vi "HandleObservationSync_003.vi"(8 "error in (no error)":errorcluster, 11 "S4GUI in":refnum<class "S4GUI.lvclass">) -> (0 "error out":errorcluster, 3 "S4GUI out":refnum<class "S4GUI.lvclass">)   [LabVIEW 2018, in "S4GUI.lvclass"] (continued)
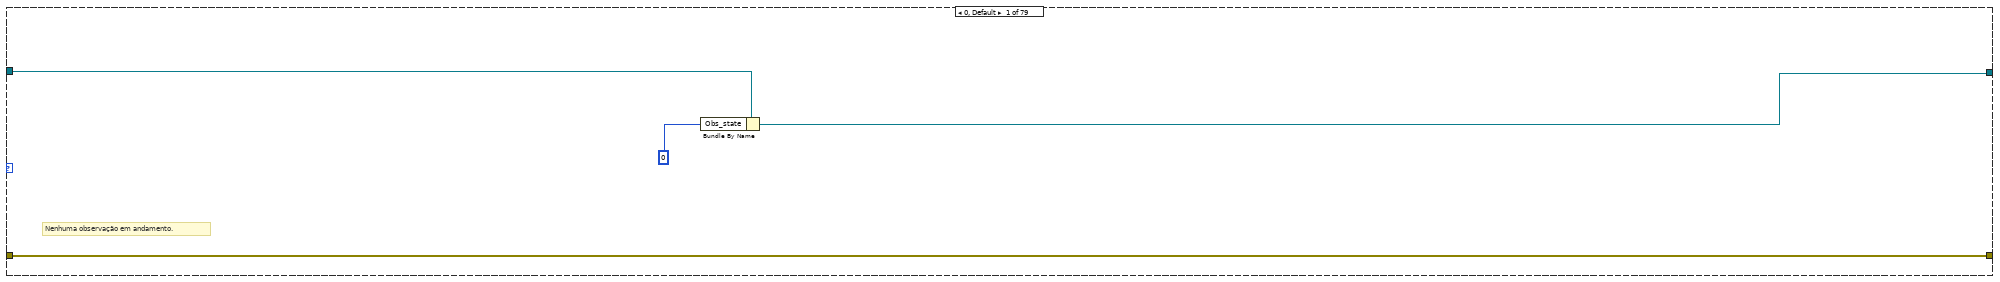
[diagram p2: hidden frame]
          n1819 = Increment(x=w5017) -> (x+1=w5016:u32)
          n1820 = Bundle By Name(cluster=w4999, "Obs_state"=w5016) -> (w5015:refnum<class "S4GUI.lvclass">)
        }
        frame 363 {
          # "T: mode EXPOSE\nF: mode FIRE\nNa seq de foco, só \ndeve usar mode EXPOSE."
          # "Espera todos os canais chegarem ao estado de repouso.\n(estado 0  de Channel:Run.vi)."
          n1821 = call-dynamic "Read AcquisitionA.vi"("error in (no error)"=w5143, "S4ACS_GUI in"=w5144) -> ("error out"=w5122:errorcluster, "Acquisition.lvclass"=w5123:refnum<class "Acquisition.lvclass">, "S4ACS_GUI out"=w5146:refnum<class "S4GUI.lvclass">)  [unwired: 7 in]
          n1822 = call-dynamic "Read enabled.vi"("error in (no error)"=w5122, "Server in"=w5123) -> ("error out"=w5124:errorcluster, "enabled"=w5126:bool, "Server out"=w5125:refnum<class "Acquisition.lvclass">)  [unwired: 7 in]
          n1823 = case shown="True" w5126 {
            tunnel: [w5220 w5238] -> w5147
            tunnel: [w5219 w5237] -> w5145
            tunnel: w5125 -> [w5220 w5230]
            tunnel: w5124 -> [w5219 w5229]
            tunnel: [TRUE w5222] -> w5103
            tunnel: [FALSE w5223] -> w5099
            frame False {
            }
            frame True {
              n1824 = call-dynamic "Read Channel.vi"("error in (no error)"=w5229, "Acquisition in"=w5230) -> ("error out"=w5226:errorcluster, "Channel.lvclass"=w5227:refnum<class "Channel.lvclass">, "Acquisition out"=w5239:refnum<class "Acquisition.lvclass">)  [unwired: 7 in]
              n1825 = call-dynamic "Read wait_expose.vi"("error in (no error)"=w5226, "Channel in"=w5227) -> ("error out"=w5224:errorcluster, "wait_expose"=w5223:bool, "Channel out"=w5225:refnum<class "Channel.lvclass">)  [unwired: 7 in]
              n1826 = call-dynamic "Read State Machine.vi"("error in (no error)"=w5224, "Device in"=w5225) -> ("error out"=w5231:errorcluster, "State Machine.lvclass"=w5233:refnum<class "State Machine.lvclass">, "Device out"=w5235:refnum<class "Channel.lvclass">)  [unwired: 7 in]
              n1827 = call-dynamic "Read State.vi"("error in (no error)"=w5231, "State Machine in"=w5233) -> ("error out"=w5228:errorcluster, "State"=w5221:i32, "State Machine out"=w5232:refnum<class "State Machine.lvclass">)  [unwired: 7 in]
              n1828 = Equal To 0?(x=w5221) -> (x = 0?=w5222:bool)
              n1829 = call-dynamic "Write State Machine.vi"("error in (no error)"=w5228, "State Machine.lvclass"=w5232, "Device in"=w5235) -> ("error out"=w5234:errorcluster, "Device out"=w5236:refnum<class "Channel.lvclass">)  [unwired: 7 in]
              n1830 = call-dynamic "Write Channel.vi"("error in (no error)"=w5234, "Channel.lvclass"=w5236, "Acquisition in"=w5239) -> ("error out"=w5237:errorcluster, "Acquisition out"=w5238:refnum<class "Acquisition.lvclass">)  [unwired: 7 in]
            }
          }
          n1831 = call-dynamic "Write AcquisitionA.vi"("error in (no error)"=w5145, "Acquisition.lvclass"=w5147, "S4ACS_GUI in"=w5146) -> ("error out"=w5139:errorcluster, "S4ACS_GUI out"=w5140:refnum<class "S4GUI.lvclass">)  [unwired: 7 in]
          n1832 = call "Read AcquisitionB.vi"("error in (no error)"=w5139, "S4ACS_GUI in"=w5140) -> ("error out"=w5119:errorcluster, "Acquisition.lvclass"=w5121:refnum<class "Acquisition.lvclass">, "S4ACS_GUI out"=w5137:refnum<class "S4GUI.lvclass">)  [unwired: 7 in]
          n1833 = call-dynamic "Read enabled.vi"("error in (no error)"=w5119, "Server in"=w5121) -> ("error out"=w5118:errorcluster, "enabled"=w5117:bool, "Server out"=w5120:refnum<class "Acquisition.lvclass">)  [unwired: 7 in]
          n1834 = case shown="True" w5117 {
            tunnel: w5120 -> [w5197 w5216]
            tunnel: w5118 -> [w5196 w5215]
            tunnel: [w5197 w5213] -> w5138
            tunnel: [w5196 w5212] -> w5136
            tunnel: [TRUE w5204] -> w5102
            tunnel: [FALSE ("expose") w5198] -> w5098
            frame False {
            }
            frame True {
              n1835 = call-dynamic "Read Channel.vi"("error in (no error)"=w5215, "Acquisition in"=w5216) -> ("error out"=w5200:errorcluster, "Channel.lvclass"=w5202:refnum<class "Channel.lvclass">, "Acquisition out"=w5214:refnum<class "Acquisition.lvclass">)  [unwired: 7 in]
              n1836 = call-dynamic "Read wait_expose.vi"("error in (no error)"=w5200, "Channel in"=w5202) -> ("error out"=w5199:errorcluster, "wait_expose"=w5198:bool, "Channel out"=w5201:refnum<class "Channel.lvclass">)  [unwired: 7 in]
              n1837 = call-dynamic "Read State Machine.vi"("error in (no error)"=w5199, "Device in"=w5201) -> ("error out"=w5206:errorcluster, "State Machine.lvclass"=w5208:refnum<class "State Machine.lvclass">, "Device out"=w5210:refnum<class "Channel.lvclass">)  [unwired: 7 in]
              n1838 = call-dynamic "Read State.vi"("error in (no error)"=w5206, "State Machine in"=w5208) -> ("error out"=w5205:errorcluster, "State"=w5203:i32, "State Machine out"=w5207:refnum<class "State Machine.lvclass">)  [unwired: 7 in]
              n1839 = Equal To 0?(x=w5203) -> (x = 0?=w5204:bool)
              n1840 = call-dynamic "Write State Machine.vi"("error in (no error)"=w5205, "State Machine.lvclass"=w5207, "Device in"=w5210) -> ("error out"=w5209:errorcluster, "Device out"=w5211:refnum<class "Channel.lvclass">)  [unwired: 7 in]
              n1841 = call-dynamic "Write Channel.vi"("error in (no error)"=w5209, "Channel.lvclass"=w5211, "Acquisition in"=w5214) -> ("error out"=w5212:errorcluster, "Acquisition out"=w5213:refnum<class "Acquisition.lvclass">)  [unwired: 7 in]
            }
          }
          n1842 = call "Write AcquisitionB.vi"("error in (no error)"=w5136, "Acquisition.lvclass"=w5138, "S4ACS_GUI in"=w5137) -> ("error out"=w5132:errorcluster, "S4ACS_GUI out"=w5131:refnum<class "S4GUI.lvclass">)  [unwired: 7 in]
          n1843 = call-dynamic "Read AcquisitionC.vi"("error in (no error)"=w5132, "S4ACS_GUI in"=w5131) -> ("error out"=w5114:errorcluster, "Acquisition.lvclass"=w5116:refnum<class "Acquisition.lvclass">, "S4ACS_GUI out"=w5134:refnum<class "S4GUI.lvclass">)  [unwired: 7 in]
          n1844 = call-dynamic "Read enabled.vi"("error in (no error)"=w5114, "Server in"=w5116) -> ("error out"=w5113:errorcluster, "enabled"=w5112:bool, "Server out"=w5115:refnum<class "Acquisition.lvclass">)  [unwired: 7 in]
          n1845 = case shown="True" w5112 {
            tunnel: [w5173 w5188] -> w5135
            tunnel: [w5174 w5187] -> w5133
            tunnel: w5115 -> [w5174 w5183]
            tunnel: w5113 -> [w5173 w5182]
            tunnel: [TRUE w5180] -> w5101
            tunnel: [FALSE ("expose") w5175] -> w5097
            frame False {
            }
            frame True {
              n1846 = call-dynamic "Read Channel.vi"("error in (no error)"=w5182, "Acquisition in"=w5183) -> ("error out"=w5177:errorcluster, "Channel.lvclass"=w5179:refnum<class "Channel.lvclass">, "Acquisition out"=w5186:refnum<class "Acquisition.lvclass">)  [unwired: 7 in]
              n1847 = call-dynamic "Read wait_expose.vi"("error in (no error)"=w5177, "Channel in"=w5179) -> ("error out"=w5176:errorcluster, "wait_expose"=w5175:bool, "Channel out"=w5178:refnum<class "Channel.lvclass">)  [unwired: 7 in]
              n1848 = call-dynamic "Read State Machine.vi"("error in (no error)"=w5176, "Device in"=w5178) -> ("error out"=w5184:errorcluster, "State Machine.lvclass"=w5192:refnum<class "State Machine.lvclass">, "Device out"=w5190:refnum<class "Channel.lvclass">)  [unwired: 7 in]
              n1849 = call-dynamic "Read State.vi"("error in (no error)"=w5184, "State Machine in"=w5192) -> ("error out"=w5185:errorcluster, "State"=w5181:i32, "State Machine out"=w5193:refnum<class "State Machine.lvclass">)  [unwired: 7 in]
              n1850 = Equal To 0?(x=w5181) -> (x = 0?=w5180:bool)
              n1851 = call-dynamic "Write State Machine.vi"("error in (no error)"=w5185, "State Machine.lvclass"=w5193, "Device in"=w5190) -> ("error out"=w5191:errorcluster, "Device out"=w5189:refnum<class "Channel.lvclass">)  [unwired: 7 in]
              n1852 = call-dynamic "Write Channel.vi"("error in (no error)"=w5191, "Channel.lvclass"=w5189, "Acquisition in"=w5186) -> ("error out"=w5188:errorcluster, "Acquisition out"=w5187:refnum<class "Acquisition.lvclass">)  [unwired: 7 in]
            }
          }
          n1853 = call-dynamic "Write AcquisitionC.vi"("error in (no error)"=w5135, "Acquisition.lvclass"=w5133, "S4ACS_GUI in"=w5134) -> ("error out"=w5111:errorcluster, "S4ACS_GUI out"=w5127:refnum<class "S4GUI.lvclass">)  [unwired: 7 in]
          n1854 = call-dynamic "Read AcquisitionD.vi"("error in (no error)"=w5111, "S4ACS_GUI in"=w5127) -> ("error out"=w5107:errorcluster, "Acquisition.lvclass"=w5110:refnum<class "Acquisition.lvclass">, "S4ACS_GUI out"=w5129:refnum<class "S4GUI.lvclass">)  [unwired: 7 in]
          n1855 = call-dynamic "Read enabled.vi"("error in (no error)"=w5107, "Server in"=w5110) -> ("error out"=w5108:errorcluster, "enabled"=w5106:bool, "Server out"=w5109:refnum<class "Acquisition.lvclass">)  [unwired: 7 in]
          n1856 = case shown="True" w5106 {
            tunnel: [w5151 w5169] -> w5130
            tunnel: [w5150 w5168] -> w5128
            tunnel: [TRUE w5158] -> w5100
            tunnel: w5109 -> [w5151 w5160]
            tunnel: w5108 -> [w5150 w5159]
            tunnel: [FALSE ("expose") w5152] -> w5096
            frame False {
            }
            frame True {
              n1857 = call-dynamic "Read Channel.vi"("error in (no error)"=w5159, "Acquisition in"=w5160) -> ("error out"=w5154:errorcluster, "Channel.lvclass"=w5156:refnum<class "Channel.lvclass">, "Acquisition out"=w5170:refnum<class "Acquisition.lvclass">)  [unwired: 7 in]
              n1858 = call-dynamic "Read wait_expose.vi"("error in (no error)"=w5154, "Channel in"=w5156) -> ("error out"=w5153:errorcluster, "wait_expose"=w5152:bool, "Channel out"=w5155:refnum<class "Channel.lvclass">)  [unwired: 7 in]
              n1859 = call-dynamic "Read State Machine.vi"("error in (no error)"=w5153, "Device in"=w5155) -> ("error out"=w5162:errorcluster, "State Machine.lvclass"=w5164:refnum<class "State Machine.lvclass">, "Device out"=w5166:refnum<class "Channel.lvclass">)  [unwired: 7 in]
              n1860 = call-dynamic "Read State.vi"("error in (no error)"=w5162, "State Machine in"=w5164) -> ("error out"=w5161:errorcluster, "State"=w5157:i32, "State Machine out"=w5163:refnum<class "State Machine.lvclass">)  [unwired: 7 in]
              n1861 = Equal To 0?(x=w5157) -> (x = 0?=w5158:bool)
              n1862 = call-dynamic "Write State Machine.vi"("error in (no error)"=w5161, "State Machine.lvclass"=w5163, "Device in"=w5166) -> ("error out"=w5165:errorcluster, "Device out"=w5167:refnum<class "Channel.lvclass">)  [unwired: 7 in]
              n1863 = call-dynamic "Write Channel.vi"("error in (no error)"=w5165, "Channel.lvclass"=w5167, "Acquisition in"=w5170) -> ("error out"=w5168:errorcluster, "Acquisition out"=w5169:refnum<class "Acquisition.lvclass">)  [unwired: 7 in]
            }
          }
          n1864 = call-dynamic "Write AcquisitionD.vi"("error in (no error)"=w5128, "Acquisition.lvclass"=w5130, "S4ACS_GUI in"=w5129) -> ("error out"=w5094:errorcluster, "S4ACS_GUI out"=w5095:refnum<class "S4GUI.lvclass">)  [unwired: 7 in]
          n1865 = Compound Arithmetic op=OR(w5099, w5098, w5097, w5096) -> ()  [unwired: 1 out]
          n1866 = Compound Arithmetic op=AND(w5103, w5102, w5101, w5100) -> (w5104:bool)
          n1867 = Increment(x=w5105) -> (x+1=w5093:u32)
          n1868 = Select(t=w5093, s=w5104, f=w5105) -> (s? t:f=w5141:u32)
          n1869 = Bundle By Name(cluster=w5095, "Obs_state"=w5141) -> (w5142:refnum<class "S4GUI.lvclass">)
        }
        frame 364 {
          n1870 = flat-sequence {
            tunnel: [w5253] -> w5241
            tunnel: w5242 -> [w5253]
            tunnel: [w5249] -> w5240
            frame #0 {
              # "Espera 2s desde que enviou o comando\nWRITE_HEADER_DATA para os ACS"
              n1871 = local read "time9"() -> (w5248:u32)
              n1872 = Tick Count (ms)() -> (millisecond timer value=w5252:u32)
              "time 10" <- w5252
              n1873 = Subtract(x=w5252, y=w5248) -> (x-y=w5251:u32)
              "delay 89" <- w5251
              n1874 = Greater?(x=w5251, y=u32 2000) -> (0:w5249:bool)
            }
          }
          n1875 = Increment(x=w5245) -> (x+1=w5244:u32)
          n1876 = Select(t=w5244, s=w5240, f=w5245) -> (s? t:f=w5246:u32)
          n1877 = Bundle By Name(cluster=w5243, "Obs_state"=w5246) -> (w5247:refnum<class "S4GUI.lvclass">)
        }
        frame 365 {
          n1878 = call-dynamic "Read AcquisitionA.vi"("error in (no error)"=w5294, "S4ACS_GUI in"=w5295) -> ("error out"=w5270:errorcluster, "Acquisition.lvclass"=w5273:refnum<class "Acquisition.lvclass">, "S4ACS_GUI out"=w5297:refnum<class "S4GUI.lvclass">)  [unwired: 7 in]
          n1879 = call-dynamic "Read enabled.vi"("error in (no error)"=w5270, "Server in"=w5273) -> ("error out"=w5269:errorcluster, "enabled"=w5271:bool, "Server out"=w5272:refnum<class "Acquisition.lvclass">)  [unwired: 7 in]
          n1880 = case shown="True" w5271 {
            tunnel: w5272 -> [w5351 w5366]
            tunnel: w5269 -> [w5350 w5365]
            tunnel: [w5351 w5363] -> w5298
            tunnel: [w5350 w5362] -> w5296
            frame False {
            }
            frame True {
              n1881 = call-dynamic "Read Channel.vi"("error in (no error)"=w5365, "Acquisition in"=w5366) -> ("error out"=w5358:errorcluster, "Channel.lvclass"=w5357:refnum<class "Channel.lvclass">, "Acquisition out"=w5364:refnum<class "Acquisition.lvclass">)  [unwired: 7 in]
              n1882 = call-dynamic "Read State Machine.vi"("error in (no error)"=w5358, "Device in"=w5357) -> ("error out"=w5359:errorcluster, "State Machine.lvclass"=w5361:refnum<class "State Machine.lvclass">, "Device out"=w5355:refnum<class "Channel.lvclass">)  [unwired: 7 in]
              n1883 = call "Next State.vi"("error in (no error)"=w5359, "New_State"=50, "State Machine in"=w5361) -> ("error out"=w5352:errorcluster, "State Machine out"=w5353:refnum<class "State Machine.lvclass">)  [unwired: 7 in]
              n1884 = call-dynamic "Write State Machine.vi"("error in (no error)"=w5352, "State Machine.lvclass"=w5353, "Device in"=w5355) -> ("error out"=w5354:errorcluster, "Device out"=w5356:refnum<class "Channel.lvclass">)  [unwired: 7 in]
              n1885 = call-dynamic "Write Channel.vi"("error in (no error)"=w5354, "Channel.lvclass"=w5356, "Acquisition in"=w5364) -> ("error out"=w5362:errorcluster, "Acquisition out"=w5363:refnum<class "Acquisition.lvclass">)  [unwired: 7 in]
            }
          }
          n1886 = call-dynamic "Write AcquisitionA.vi"("error in (no error)"=w5296, "Acquisition.lvclass"=w5298, "S4ACS_GUI in"=w5297) -> ("error out"=w5289:errorcluster, "S4ACS_GUI out"=w5290:refnum<class "S4GUI.lvclass">)  [unwired: 7 in]
          n1887 = call "Read AcquisitionB.vi"("error in (no error)"=w5289, "S4ACS_GUI in"=w5290) -> ("error out"=w5266:errorcluster, "Acquisition.lvclass"=w5268:refnum<class "Acquisition.lvclass">, "S4ACS_GUI out"=w5287:refnum<class "S4GUI.lvclass">)  [unwired: 7 in]
          n1888 = call-dynamic "Read enabled.vi"("error in (no error)"=w5266, "Server in"=w5268) -> ("error out"=w5265:errorcluster, "enabled"=w5264:bool, "Server out"=w5267:refnum<class "Acquisition.lvclass">)  [unwired: 7 in]
          n1889 = case shown="True" w5264 {
            tunnel: w5267 -> [w5334 w5349]
            tunnel: w5265 -> [w5333 w5348]
            tunnel: [w5334 w5346] -> w5288
            tunnel: [w5333 w5345] -> w5286
            frame False {
            }
            frame True {
              n1890 = call-dynamic "Read Channel.vi"("error in (no error)"=w5348, "Acquisition in"=w5349) -> ("error out"=w5341:errorcluster, "Channel.lvclass"=w5340:refnum<class "Channel.lvclass">, "Acquisition out"=w5347:refnum<class "Acquisition.lvclass">)  [unwired: 7 in]
              n1891 = call-dynamic "Read State Machine.vi"("error in (no error)"=w5341, "Device in"=w5340) -> ("error out"=w5342:errorcluster, "State Machine.lvclass"=w5344:refnum<class "State Machine.lvclass">, "Device out"=w5338:refnum<class "Channel.lvclass">)  [unwired: 7 in]
              n1892 = call "Next State.vi"("error in (no error)"=w5342, "New_State"=50, "State Machine in"=w5344) -> ("error out"=w5335:errorcluster, "State Machine out"=w5336:refnum<class "State Machine.lvclass">)  [unwired: 7 in]
              n1893 = call-dynamic "Write State Machine.vi"("error in (no error)"=w5335, "State Machine.lvclass"=w5336, "Device in"=w5338) -> ("error out"=w5337:errorcluster, "Device out"=w5339:refnum<class "Channel.lvclass">)  [unwired: 7 in]
              n1894 = call-dynamic "Write Channel.vi"("error in (no error)"=w5337, "Channel.lvclass"=w5339, "Acquisition in"=w5347) -> ("error out"=w5345:errorcluster, "Acquisition out"=w5346:refnum<class "Acquisition.lvclass">)  [unwired: 7 in]
            }
          }
          n1895 = call "Write AcquisitionB.vi"("error in (no error)"=w5286, "Acquisition.lvclass"=w5288, "S4ACS_GUI in"=w5287) -> ("error out"=w5282:errorcluster, "S4ACS_GUI out"=w5281:refnum<class "S4GUI.lvclass">)  [unwired: 7 in]
          n1896 = call-dynamic "Read AcquisitionC.vi"("error in (no error)"=w5282, "S4ACS_GUI in"=w5281) -> ("error out"=w5261:errorcluster, "Acquisition.lvclass"=w5263:refnum<class "Acquisition.lvclass">, "S4ACS_GUI out"=w5284:refnum<class "S4GUI.lvclass">)  [unwired: 7 in]
          n1897 = call-dynamic "Read enabled.vi"("error in (no error)"=w5261, "Server in"=w5263) -> ("error out"=w5260:errorcluster, "enabled"=w5259:bool, "Server out"=w5262:refnum<class "Acquisition.lvclass">)  [unwired: 7 in]
          n1898 = case shown="True" w5259 {
            tunnel: [w5316 w5324] -> w5285
            tunnel: [w5317 w5323] -> w5283
            tunnel: w5262 -> [w5317 w5321]
            tunnel: w5260 -> [w5316 w5320]
            frame False {
            }
            frame True {
              n1899 = call-dynamic "Read Channel.vi"("error in (no error)"=w5320, "Acquisition in"=w5321) -> ("error out"=w5328:errorcluster, "Channel.lvclass"=w5329:refnum<class "Channel.lvclass">, "Acquisition out"=w5322:refnum<class "Acquisition.lvclass">)  [unwired: 7 in]
              n1900 = call-dynamic "Read State Machine.vi"("error in (no error)"=w5328, "Device in"=w5329) -> ("error out"=w5327:errorcluster, "State Machine.lvclass"=w5325:refnum<class "State Machine.lvclass">, "Device out"=w5331:refnum<class "Channel.lvclass">)  [unwired: 7 in]
              n1901 = call "Next State.vi"("error in (no error)"=w5327, "New_State"=50, "State Machine in"=w5325) -> ("error out"=w5319:errorcluster, "State Machine out"=w5318:refnum<class "State Machine.lvclass">)  [unwired: 7 in]
              n1902 = call-dynamic "Write State Machine.vi"("error in (no error)"=w5319, "State Machine.lvclass"=w5318, "Device in"=w5331) -> ("error out"=w5332:errorcluster, "Device out"=w5330:refnum<class "Channel.lvclass">)  [unwired: 7 in]
              n1903 = call-dynamic "Write Channel.vi"("error in (no error)"=w5332, "Channel.lvclass"=w5330, "Acquisition in"=w5322) -> ("error out"=w5324:errorcluster, "Acquisition out"=w5323:refnum<class "Acquisition.lvclass">)  [unwired: 7 in]
            }
          }
          n1904 = call-dynamic "Write AcquisitionC.vi"("error in (no error)"=w5285, "Acquisition.lvclass"=w5283, "S4ACS_GUI in"=w5284) -> ("error out"=w5279:errorcluster, "S4ACS_GUI out"=w5278:refnum<class "S4GUI.lvclass">)  [unwired: 7 in]
          n1905 = call-dynamic "Read AcquisitionD.vi"("error in (no error)"=w5279, "S4ACS_GUI in"=w5278) -> ("error out"=w5256:errorcluster, "Acquisition.lvclass"=w5258:refnum<class "Acquisition.lvclass">, "S4ACS_GUI out"=w5277:refnum<class "S4GUI.lvclass">)  [unwired: 7 in]
          n1906 = call-dynamic "Read enabled.vi"("error in (no error)"=w5256, "Server in"=w5258) -> ("error out"=w5255:errorcluster, "enabled"=w5254:bool, "Server out"=w5257:refnum<class "Acquisition.lvclass">)  [unwired: 7 in]
          n1907 = case shown="True" w5254 {
            tunnel: w5255 -> [w5299 w5315]
            tunnel: [w5299 w5314] -> w5280
            tunnel: w5257 -> [w5300 w5305]
            tunnel: [w5300 w5303] -> w5276
            frame False {
            }
            frame True {
              n1908 = call-dynamic "Read Channel.vi"("error in (no error)"=w5315, "Acquisition in"=w5305) -> ("error out"=w5310:errorcluster, "Channel.lvclass"=w5309:refnum<class "Channel.lvclass">, "Acquisition out"=w5304:refnum<class "Acquisition.lvclass">)  [unwired: 7 in]
              n1909 = call-dynamic "Read State Machine.vi"("error in (no error)"=w5310, "Device in"=w5309) -> ("error out"=w5311:errorcluster, "State Machine.lvclass"=w5313:refnum<class "State Machine.lvclass">, "Device out"=w5307:refnum<class "Channel.lvclass">)  [unwired: 7 in]
              n1910 = call "Next State.vi"("error in (no error)"=w5311, "New_State"=50, "State Machine in"=w5313) -> ("error out"=w5301:errorcluster, "State Machine out"=w5302:refnum<class "State Machine.lvclass">)  [unwired: 7 in]
              n1911 = call-dynamic "Write State Machine.vi"("error in (no error)"=w5301, "State Machine.lvclass"=w5302, "Device in"=w5307) -> ("error out"=w5306:errorcluster, "Device out"=w5308:refnum<class "Channel.lvclass">)  [unwired: 7 in]
              n1912 = call-dynamic "Write Channel.vi"("error in (no error)"=w5306, "Channel.lvclass"=w5308, "Acquisition in"=w5304) -> ("error out"=w5314:errorcluster, "Acquisition out"=w5303:refnum<class "Acquisition.lvclass">)  [unwired: 7 in]
            }
          }
          n1913 = call-dynamic "Write AcquisitionD.vi"("error in (no error)"=w5280, "Acquisition.lvclass"=w5276, "S4ACS_GUI in"=w5277) -> ("error out"=w5275:errorcluster, "S4ACS_GUI out"=w5274:refnum<class "S4GUI.lvclass">)  [unwired: 7 in]
          n1914 = Increment(x=w5293) -> (x+1=w5292:u32)
          n1915 = Bundle By Name(cluster=w5274, "Obs_state"=w5292) -> (w5291:refnum<class "S4GUI.lvclass">)
        }
        frame 366 {
          # "Espera todos os canais com CyclesDone=0"
          # "Espera todos os canais chegarem ao estado ACTIVE\n(estados 54 e 55 de Channel:Run.vi)."
          n1916 = call-dynamic "Read AcquisitionA.vi"("error in (no error)"=w5418, "S4ACS_GUI in"=w5419) -> ("error out"=w5397:errorcluster, "Acquisition.lvclass"=w5398:refnum<class "Acquisition.lvclass">, "S4ACS_GUI out"=w5421:refnum<class "S4GUI.lvclass">)  [unwired: 7 in]
          n1917 = call-dynamic "Read enabled.vi"("error in (no error)"=w5397, "Server in"=w5398) -> ("error out"=w5399:errorcluster, "enabled"=w5401:bool, "Server out"=w5400:refnum<class "Acquisition.lvclass">)  [unwired: 7 in]
          n1918 = case shown="True" w5401 {
            tunnel: [w5498 w5517] -> w5422
            tunnel: [w5497 w5516] -> w5420
            tunnel: w5400 -> [w5498 w5509]
            tunnel: w5399 -> [w5497 w5508]
            tunnel: [TRUE w5507] -> w5379
            tunnel: [u32 0 ("CyclesDone") w5499] -> w5371
            frame False {
            }
            frame True {
              n1919 = call-dynamic "Read Channel.vi"("error in (no error)"=w5508, "Acquisition in"=w5509) -> ("error out"=w5502:errorcluster, "Channel.lvclass"=w5503:refnum<class "Channel.lvclass">, "Acquisition out"=w5518:refnum<class "Acquisition.lvclass">)  [unwired: 7 in]
              n1920 = call-dynamic "Read CyclesDone.vi"("error in (no error)"=w5502, "Channel in"=w5503) -> ("error out"=w5500:errorcluster, "CyclesDone"=w5499:u32, "Channel out"=w5501:refnum<class "Channel.lvclass">)  [unwired: 7 in]
              n1921 = call-dynamic "Read State Machine.vi"("error in (no error)"=w5500, "Device in"=w5501) -> ("error out"=w5510:errorcluster, "State Machine.lvclass"=w5512:refnum<class "State Machine.lvclass">, "Device out"=w5514:refnum<class "Channel.lvclass">)  [unwired: 7 in]
              n1922 = call-dynamic "Read State.vi"("error in (no error)"=w5510, "State Machine in"=w5512) -> ("error out"=w5504:errorcluster, "State"=w5506:i32, "State Machine out"=w5511:refnum<class "State Machine.lvclass">)  [unwired: 7 in]
              n1923 = Greater?(x=w5506, y=53) -> (0:w5507:bool)
              n1924 = call-dynamic "Write State Machine.vi"("error in (no error)"=w5504, "State Machine.lvclass"=w5511, "Device in"=w5514) -> ("error out"=w5513:errorcluster, "Device out"=w5515:refnum<class "Channel.lvclass">)  [unwired: 7 in]
              n1925 = call-dynamic "Write Channel.vi"("error in (no error)"=w5513, "Channel.lvclass"=w5515, "Acquisition in"=w5518) -> ("error out"=w5516:errorcluster, "Acquisition out"=w5517:refnum<class "Acquisition.lvclass">)  [unwired: 7 in]
            }
          }
          n1926 = call-dynamic "Write AcquisitionA.vi"("error in (no error)"=w5420, "Acquisition.lvclass"=w5422, "S4ACS_GUI in"=w5421) -> ("error out"=w5414:errorcluster, "S4ACS_GUI out"=w5415:refnum<class "S4GUI.lvclass">)  [unwired: 7 in]
          n1927 = call "Read AcquisitionB.vi"("error in (no error)"=w5414, "S4ACS_GUI in"=w5415) -> ("error out"=w5394:errorcluster, "Acquisition.lvclass"=w5396:refnum<class "Acquisition.lvclass">, "S4ACS_GUI out"=w5412:refnum<class "S4GUI.lvclass">)  [unwired: 7 in]
          n1928 = call-dynamic "Read enabled.vi"("error in (no error)"=w5394, "Server in"=w5396) -> ("error out"=w5393:errorcluster, "enabled"=w5392:bool, "Server out"=w5395:refnum<class "Acquisition.lvclass">)  [unwired: 7 in]
          n1929 = case shown="True" w5392 {
            tunnel: w5395 -> [w5474 w5494]
            tunnel: w5393 -> [w5473 w5493]
            tunnel: [w5474 w5491] -> w5413
            tunnel: [w5473 w5490] -> w5411
            tunnel: [TRUE w5481] -> w5378
            tunnel: [u32 0 ("CyclesDone") w5475] -> w5372
            frame False {
            }
            frame True {
              n1930 = call-dynamic "Read Channel.vi"("error in (no error)"=w5493, "Acquisition in"=w5494) -> ("error out"=w5477:errorcluster, "Channel.lvclass"=w5479:refnum<class "Channel.lvclass">, "Acquisition out"=w5492:refnum<class "Acquisition.lvclass">)  [unwired: 7 in]
              n1931 = call-dynamic "Read CyclesDone.vi"("error in (no error)"=w5477, "Channel in"=w5479) -> ("error out"=w5476:errorcluster, "CyclesDone"=w5475:u32, "Channel out"=w5478:refnum<class "Channel.lvclass">)  [unwired: 7 in]
              n1932 = call-dynamic "Read State Machine.vi"("error in (no error)"=w5476, "Device in"=w5478) -> ("error out"=w5484:errorcluster, "State Machine.lvclass"=w5486:refnum<class "State Machine.lvclass">, "Device out"=w5488:refnum<class "Channel.lvclass">)  [unwired: 7 in]
              n1933 = call-dynamic "Read State.vi"("error in (no error)"=w5484, "State Machine in"=w5486) -> ("error out"=w5483:errorcluster, "State"=w5480:i32, "State Machine out"=w5485:refnum<class "State Machine.lvclass">)  [unwired: 7 in]
              n1934 = Greater?(x=w5480, y=53) -> (0:w5481:bool)
              n1935 = call-dynamic "Write State Machine.vi"("error in (no error)"=w5483, "State Machine.lvclass"=w5485, "Device in"=w5488) -> ("error out"=w5487:errorcluster, "Device out"=w5489:refnum<class "Channel.lvclass">)  [unwired: 7 in]
              n1936 = call-dynamic "Write Channel.vi"("error in (no error)"=w5487, "Channel.lvclass"=w5489, "Acquisition in"=w5492) -> ("error out"=w5490:errorcluster, "Acquisition out"=w5491:refnum<class "Acquisition.lvclass">)  [unwired: 7 in]
            }
          }
          n1937 = call "Write AcquisitionB.vi"("error in (no error)"=w5411, "Acquisition.lvclass"=w5413, "S4ACS_GUI in"=w5412) -> ("error out"=w5407:errorcluster, "S4ACS_GUI out"=w5406:refnum<class "S4GUI.lvclass">)  [unwired: 7 in]
          n1938 = call-dynamic "Read AcquisitionC.vi"("error in (no error)"=w5407, "S4ACS_GUI in"=w5406) -> ("error out"=w5389:errorcluster, "Acquisition.lvclass"=w5391:refnum<class "Acquisition.lvclass">, "S4ACS_GUI out"=w5409:refnum<class "S4GUI.lvclass">)  [unwired: 7 in]
          n1939 = call-dynamic "Read enabled.vi"("error in (no error)"=w5389, "Server in"=w5391) -> ("error out"=w5388:errorcluster, "enabled"=w5387:bool, "Server out"=w5390:refnum<class "Acquisition.lvclass">)  [unwired: 7 in]
          n1940 = case shown="True" w5387 {
            tunnel: [w5449 w5465] -> w5410
            tunnel: [w5450 w5464] -> w5408
            tunnel: w5390 -> [w5450 w5460]
            tunnel: w5388 -> [w5449 w5459]
            tunnel: [TRUE w5456] -> w5377
            tunnel: [u32 0 ("CyclesDone") w5451] -> w5370
            frame False {
            }
            frame True {
              n1941 = call-dynamic "Read Channel.vi"("error in (no error)"=w5459, "Acquisition in"=w5460) -> ("error out"=w5453:errorcluster, "Channel.lvclass"=w5455:refnum<class "Channel.lvclass">, "Acquisition out"=w5463:refnum<class "Acquisition.lvclass">)  [unwired: 7 in]
              n1942 = call-dynamic "Read CyclesDone.vi"("error in (no error)"=w5453, "Channel in"=w5455) -> ("error out"=w5452:errorcluster, "CyclesDone"=w5451:u32, "Channel out"=w5454:refnum<class "Channel.lvclass">)  [unwired: 7 in]
              n1943 = call-dynamic "Read State Machine.vi"("error in (no error)"=w5452, "Device in"=w5454) -> ("error out"=w5461:errorcluster, "State Machine.lvclass"=w5469:refnum<class "State Machine.lvclass">, "Device out"=w5467:refnum<class "Channel.lvclass">)  [unwired: 7 in]
              n1944 = call-dynamic "Read State.vi"("error in (no error)"=w5461, "State Machine in"=w5469) -> ("error out"=w5462:errorcluster, "State"=w5457:i32, "State Machine out"=w5470:refnum<class "State Machine.lvclass">)  [unwired: 7 in]
              n1945 = Greater?(x=w5457, y=53) -> (0:w5456:bool)
              n1946 = call-dynamic "Write State Machine.vi"("error in (no error)"=w5462, "State Machine.lvclass"=w5470, "Device in"=w5467) -> ("error out"=w5468:errorcluster, "Device out"=w5466:refnum<class "Channel.lvclass">)  [unwired: 7 in]
              n1947 = call-dynamic "Write Channel.vi"("error in (no error)"=w5468, "Channel.lvclass"=w5466, "Acquisition in"=w5463) -> ("error out"=w5465:errorcluster, "Acquisition out"=w5464:refnum<class "Acquisition.lvclass">)  [unwired: 7 in]
            }
          }
          n1948 = call-dynamic "Write AcquisitionC.vi"("error in (no error)"=w5410, "Acquisition.lvclass"=w5408, "S4ACS_GUI in"=w5409) -> ("error out"=w5386:errorcluster, "S4ACS_GUI out"=w5402:refnum<class "S4GUI.lvclass">)  [unwired: 7 in]
          n1949 = call-dynamic "Read AcquisitionD.vi"("error in (no error)"=w5386, "S4ACS_GUI in"=w5402) -> ("error out"=w5382:errorcluster, "Acquisition.lvclass"=w5385:refnum<class "Acquisition.lvclass">, "S4ACS_GUI out"=w5404:refnum<class "S4GUI.lvclass">)  [unwired: 7 in]
          n1950 = call-dynamic "Read enabled.vi"("error in (no error)"=w5382, "Server in"=w5385) -> ("error out"=w5383:errorcluster, "enabled"=w5381:bool, "Server out"=w5384:refnum<class "Acquisition.lvclass">)  [unwired: 7 in]
          n1951 = case shown="True" w5381 {
            tunnel: [w5426 w5445] -> w5405
            tunnel: [w5425 w5444] -> w5403
            tunnel: [TRUE w5433] -> w5376
            tunnel: w5384 -> [w5426 w5436]
            tunnel: w5383 -> [w5425 w5435]
            tunnel: [u32 0 ("CyclesDone") w5427] -> w5369
            frame False {
            }
            frame True {
              n1952 = call-dynamic "Read Channel.vi"("error in (no error)"=w5435, "Acquisition in"=w5436) -> ("error out"=w5429:errorcluster, "Channel.lvclass"=w5431:refnum<class "Channel.lvclass">, "Acquisition out"=w5446:refnum<class "Acquisition.lvclass">)  [unwired: 7 in]
              n1953 = call-dynamic "Read CyclesDone.vi"("error in (no error)"=w5429, "Channel in"=w5431) -> ("error out"=w5428:errorcluster, "CyclesDone"=w5427:u32, "Channel out"=w5430:refnum<class "Channel.lvclass">)  [unwired: 7 in]
              n1954 = call-dynamic "Read State Machine.vi"("error in (no error)"=w5428, "Device in"=w5430) -> ("error out"=w5438:errorcluster, "State Machine.lvclass"=w5440:refnum<class "State Machine.lvclass">, "Device out"=w5442:refnum<class "Channel.lvclass">)  [unwired: 7 in]
              n1955 = call-dynamic "Read State.vi"("error in (no error)"=w5438, "State Machine in"=w5440) -> ("error out"=w5437:errorcluster, "State"=w5432:i32, "State Machine out"=w5439:refnum<class "State Machine.lvclass">)  [unwired: 7 in]
              n1956 = Greater?(x=w5432, y=53) -> (0:w5433:bool)
              n1957 = call-dynamic "Write State Machine.vi"("error in (no error)"=w5437, "State Machine.lvclass"=w5439, "Device in"=w5442) -> ("error out"=w5441:errorcluster, "Device out"=w5443:refnum<class "Channel.lvclass">)  [unwired: 7 in]
              n1958 = call-dynamic "Write Channel.vi"("error in (no error)"=w5441, "Channel.lvclass"=w5443, "Acquisition in"=w5446) -> ("error out"=w5444:errorcluster, "Acquisition out"=w5445:refnum<class "Acquisition.lvclass">)  [unwired: 7 in]
            }
          }
          n1959 = call-dynamic "Write AcquisitionD.vi"("error in (no error)"=w5403, "Acquisition.lvclass"=w5405, "S4ACS_GUI in"=w5404) -> ("error out"=w5374:errorcluster, "S4ACS_GUI out"=w5375:refnum<class "S4GUI.lvclass">)  [unwired: 7 in]
          n1960 = Compound Arithmetic op=AND(w5379, w5378, w5377, w5376) -> ()  [unwired: 1 out]
          n1961 = Compound Arithmetic op=ADD(w5371, w5372, w5370, w5369) -> (w5368:u32)
          n1962 = Equal To 0?(x=w5368) -> (x = 0?=w5367:bool)
          n1963 = Increment(x=w5380) -> (x+1=w5373:u32)
          n1964 = Select(t=w5373, s=w5367, f=w5380) -> (s? t:f=w5416:u32)
          n1965 = Bundle By Name(cluster=w5375, "Obs_state"=w5416) -> (w5417:refnum<class "S4GUI.lvclass">)
        }
        frame 367 {
          # "T=canais receberam STOP"
          # "OV 2024.01.26 DEBUG - ignora os ciclos!!\nT= Todos os canais ativos no mesmo ciclo;\nF= Canais com ciclo diferente"
          # "T= Todos os canais ativos na mesma sequencia;\nF= Canais com sequencia diferente"
          # "Todos os CYCLES_DONE \nmudaram e são iguais?\nSe sim, avança a lâmina."
          n1966 = Unbundle By Name(w5554) -> ("cyclesDone"=w5548:u32)
          n1967 = call-dynamic "Read AcquisitionA.vi"("error in (no error)"=w5589, "S4ACS_GUI in"=w5554) -> ("error out"=w5569:errorcluster, "Acquisition.lvclass"=w5570:refnum<class "Acquisition.lvclass">, "S4ACS_GUI out"=w5591:refnum<class "S4GUI.lvclass">)  [unwired: 7 in]
          n1968 = call-dynamic "Read enabled.vi"("error in (no error)"=w5569, "Server in"=w5570) -> ("error out"=w5568:errorcluster, "enabled"=w5536:bool, "Server out"=w5567:refnum<class "Acquisition.lvclass">)  [unwired: 7 in]
          n1969 = case shown="True" w5536 {
            tunnel: w5568 -> [w5806 w5825]
            tunnel: [w5807 w5823] -> w5592
            tunnel: [w5806 w5822] -> w5590
            tunnel: [u32 0 ("SequesDone") w5821] -> w5542
            tunnel: w5567 -> [w5807 w5820]
            tunnel: w5548 -> [_ w5819]
            tunnel: [TRUE w5818] -> w5553
            tunnel: [u32 0 ("CubesDone") w5817] -> w5529
            tunnel: [FALSE ("stopping") w5808] -> w5525
            frame False {
            }
            frame True {
              # "CYCLES_DONE = 0->1"
              n1970 = call-dynamic "Read Channel.vi"("error in (no error)"=w5825, "Acquisition in"=w5820) -> ("error out"=w5814:errorcluster, "Channel.lvclass"=w5816:refnum<class "Channel.lvclass">, "Acquisition out"=w5824:refnum<class "Acquisition.lvclass">)  [unwired: 7 in]
              n1971 = call-dynamic "Read CyclesDone.vi"("error in (no error)"=w5814, "Channel in"=w5816) -> ("error out"=w5813:errorcluster, "CyclesDone"=w5817:u32, "Channel out"=w5815:refnum<class "Channel.lvclass">)  [unwired: 7 in]
              n1972 = call-dynamic "Read CyclesDone.vi"("error in (no error)"=w5813, "Channel in"=w5815) -> ("error out"=w5811:errorcluster, "CyclesDone"=w5821:u32, "Channel out"=w5812:refnum<class "Channel.lvclass">)  [unwired: 7 in]
              n1973 = Not Equal?(x=w5821, y=w5819) -> (x != y?=w5818:bool)
              n1974 = call-dynamic "Read stopping.vi"("error in (no error)"=w5811, "Channel in"=w5812) -> ("error out"=w5810:errorcluster, "stopping"=w5808:bool, "Channel out"=w5809:refnum<class "Channel.lvclass">)  [unwired: 7 in]
              n1975 = call-dynamic "Write Channel.vi"("error in (no error)"=w5810, "Channel.lvclass"=w5809, "Acquisition in"=w5824) -> ("error out"=w5822:errorcluster, "Acquisition out"=w5823:refnum<class "Acquisition.lvclass">)  [unwired: 7 in]
            }
          }
          n1976 = call-dynamic "Write AcquisitionA.vi"("error in (no error)"=w5590, "Acquisition.lvclass"=w5592, "S4ACS_GUI in"=w5591) -> ("error out"=w5586:errorcluster, "S4ACS_GUI out"=w5585:refnum<class "S4GUI.lvclass">)  [unwired: 7 in]
          n1977 = call "Read AcquisitionB.vi"("error in (no error)"=w5586, "S4ACS_GUI in"=w5585) -> ("error out"=w5563:errorcluster, "Acquisition.lvclass"=w5566:refnum<class "Acquisition.lvclass">, "S4ACS_GUI out"=w5587:refnum<class "S4GUI.lvclass">)  [unwired: 7 in]
          n1978 = call-dynamic "Read enabled.vi"("error in (no error)"=w5563, "Server in"=w5566) -> ("error out"=w5564:errorcluster, "enabled"=w5535:bool, "Server out"=w5565:refnum<class "Acquisition.lvclass">)  [unwired: 7 in]
          n1979 = case shown="True" w5535 {
            tunnel: w5564 -> [w5782 w5801]
            tunnel: w5565 -> [w5783 w5800]
            tunnel: [u32 0 ("SequesDone") w5795] -> w5539
            tunnel: [w5782 w5799] -> w5584
            tunnel: [w5783 w5798] -> w5583
            tunnel: w5548 -> [_ w5794]
            tunnel: [TRUE w5793] -> w5549
            tunnel: [u32 0 ("CubesDone") w5788] -> w5528
            tunnel: [FALSE ("stopping") w5784] -> w5524
            frame False {
            }
            frame True {
              n1980 = call-dynamic "Read Channel.vi"("error in (no error)"=w5801, "Acquisition in"=w5800) -> ("error out"=w5790:errorcluster, "Channel.lvclass"=w5792:refnum<class "Channel.lvclass">, "Acquisition out"=w5796:refnum<class "Acquisition.lvclass">)  [unwired: 7 in]
              n1981 = call-dynamic "Read CyclesDone.vi"("error in (no error)"=w5790, "Channel in"=w5792) -> ("error out"=w5789:errorcluster, "CyclesDone"=w5788:u32, "Channel out"=w5791:refnum<class "Channel.lvclass">)  [unwired: 7 in]
              n1982 = call-dynamic "Read CyclesDone.vi"("error in (no error)"=w5789, "Channel in"=w5791) -> ("error out"=w5786:errorcluster, "CyclesDone"=w5795:u32, "Channel out"=w5797:refnum<class "Channel.lvclass">)  [unwired: 7 in]
              n1983 = Not Equal?(x=w5795, y=w5794) -> (x != y?=w5793:bool)
              n1984 = call-dynamic "Read stopping.vi"("error in (no error)"=w5786, "Channel in"=w5797) -> ("error out"=w5785:errorcluster, "stopping"=w5784:bool, "Channel out"=w5787:refnum<class "Channel.lvclass">)  [unwired: 7 in]
              n1985 = call-dynamic "Write Channel.vi"("error in (no error)"=w5785, "Channel.lvclass"=w5787, "Acquisition in"=w5796) -> ("error out"=w5799:errorcluster, "Acquisition out"=w5798:refnum<class "Acquisition.lvclass">)  [unwired: 7 in]
            }
          }
          n1986 = Max & Min(x=w5529, y=w5528) -> (max(x,y)=w5545:u32)  [unwired: 1 out]
          n1987 = Max & Min(x=w5542, y=w5539) -> (max(x,y)=w5552:u32)  [unwired: 1 out]
          n1988 = call "Write AcquisitionB.vi"("error in (no error)"=w5584, "Acquisition.lvclass"=w5583, "S4ACS_GUI in"=w5587) -> ("error out"=w5576:errorcluster, "S4ACS_GUI out"=w5575:refnum<class "S4GUI.lvclass">)  [unwired: 7 in]
          n1989 = call-dynamic "Read AcquisitionC.vi"("error in (no error)"=w5576, "S4ACS_GUI in"=w5575) -> ("error out"=w5560:errorcluster, "Acquisition.lvclass"=w5562:refnum<class "Acquisition.lvclass">, "S4ACS_GUI out"=w5578:refnum<class "S4GUI.lvclass">)  [unwired: 7 in]
          n1990 = call-dynamic "Read enabled.vi"("error in (no error)"=w5560, "Server in"=w5562) -> ("error out"=w5559:errorcluster, "enabled"=w5534:bool, "Server out"=w5561:refnum<class "Acquisition.lvclass">)  [unwired: 7 in]
          n1991 = case shown="True" w5534 {
            tunnel: [w5758 w5777] -> w5579
            tunnel: [w5759 w5776] -> w5577
            tunnel: w5559 -> [w5758 w5773]
            tunnel: w5561 -> [w5759 w5774]
            tunnel: [u32 0 ("SequesDone") w5772] -> w5538
            tunnel: w5548 -> [_ w5771]
            tunnel: [TRUE w5770] -> w5547
            tunnel: [u32 0 ("CubesDone") w5764] -> w5527
            tunnel: [FALSE ("stopping") w5760] -> w5523
            frame False {
            }
            frame True {
              n1992 = call-dynamic "Read Channel.vi"("error in (no error)"=w5773, "Acquisition in"=w5774) -> ("error out"=w5766:errorcluster, "Channel.lvclass"=w5768:refnum<class "Channel.lvclass">, "Acquisition out"=w5775:refnum<class "Acquisition.lvclass">)  [unwired: 7 in]
              n1993 = call-dynamic "Read CyclesDone.vi"("error in (no error)"=w5766, "Channel in"=w5768) -> ("error out"=w5765:errorcluster, "CyclesDone"=w5764:u32, "Channel out"=w5767:refnum<class "Channel.lvclass">)  [unwired: 7 in]
              n1994 = call-dynamic "Read CyclesDone.vi"("error in (no error)"=w5765, "Channel in"=w5767) -> ("error out"=w5762:errorcluster, "CyclesDone"=w5772:u32, "Channel out"=w5769:refnum<class "Channel.lvclass">)  [unwired: 7 in]
              n1995 = Not Equal?(x=w5772, y=w5771) -> (x != y?=w5770:bool)
              n1996 = call-dynamic "Read stopping.vi"("error in (no error)"=w5762, "Channel in"=w5769) -> ("error out"=w5761:errorcluster, "stopping"=w5760:bool, "Channel out"=w5763:refnum<class "Channel.lvclass">)  [unwired: 7 in]
              n1997 = call-dynamic "Write Channel.vi"("error in (no error)"=w5761, "Channel.lvclass"=w5763, "Acquisition in"=w5775) -> ("error out"=w5777:errorcluster, "Acquisition out"=w5776:refnum<class "Acquisition.lvclass">)  [unwired: 7 in]
            }
          }
          n1998 = call-dynamic "Write AcquisitionC.vi"("error in (no error)"=w5579, "Acquisition.lvclass"=w5577, "S4ACS_GUI in"=w5578) -> ("error out"=w5573:errorcluster, "S4ACS_GUI out"=w5574:refnum<class "S4GUI.lvclass">)  [unwired: 7 in]
          n1999 = call-dynamic "Read AcquisitionD.vi"("error in (no error)"=w5573, "S4ACS_GUI in"=w5574) -> ("error out"=w5556:errorcluster, "Acquisition.lvclass"=w5558:refnum<class "Acquisition.lvclass">, "S4ACS_GUI out"=w5580:refnum<class "S4GUI.lvclass">)  [unwired: 7 in]
          n2000 = call-dynamic "Read enabled.vi"("error in (no error)"=w5556, "Server in"=w5558) -> ("error out"=w5555:errorcluster, "enabled"=w5533:bool, "Server out"=w5557:refnum<class "Acquisition.lvclass">)  [unwired: 7 in]
          n2001 = Build Array(w5536, w5535, w5534, w5533) -> (w5532:bool[])
          n2002 = case shown="True" w5533 {
            tunnel: [w5735 w5753] -> w5582
            tunnel: [w5734 w5752] -> w5581
            tunnel: w5557 -> [w5735 w5751]
            tunnel: w5555 -> [w5734 w5750]
            tunnel: [u32 0 ("SequesDone") w5748] -> w5541
            tunnel: w5548 -> [_ w5747]
            tunnel: [TRUE w5746] -> w5546
            tunnel: [u32 0 ("CubesDone") w5740] -> w5526
            tunnel: [FALSE ("stopping") w5736] -> w5522
            frame False {
            }
            frame True {
              n2003 = call-dynamic "Read Channel.vi"("error in (no error)"=w5750, "Acquisition in"=w5751) -> ("error out"=w5742:errorcluster, "Channel.lvclass"=w5744:refnum<class "Channel.lvclass">, "Acquisition out"=w5749:refnum<class "Acquisition.lvclass">)  [unwired: 7 in]
              n2004 = call-dynamic "Read CyclesDone.vi"("error in (no error)"=w5742, "Channel in"=w5744) -> ("error out"=w5741:errorcluster, "CyclesDone"=w5740:u32, "Channel out"=w5743:refnum<class "Channel.lvclass">)  [unwired: 7 in]
              n2005 = call-dynamic "Read CyclesDone.vi"("error in (no error)"=w5741, "Channel in"=w5743) -> ("error out"=w5738:errorcluster, "CyclesDone"=w5748:u32, "Channel out"=w5745:refnum<class "Channel.lvclass">)  [unwired: 7 in]
              n2006 = Not Equal?(x=w5748, y=w5747) -> (x != y?=w5746:bool)
              n2007 = call-dynamic "Read stopping.vi"("error in (no error)"=w5738, "Channel in"=w5745) -> ("error out"=w5737:errorcluster, "stopping"=w5736:bool, "Channel out"=w5739:refnum<class "Channel.lvclass">)  [unwired: 7 in]
              n2008 = call-dynamic "Write Channel.vi"("error in (no error)"=w5737, "Channel.lvclass"=w5739, "Acquisition in"=w5749) -> ("error out"=w5752:errorcluster, "Acquisition out"=w5753:refnum<class "Acquisition.lvclass">)  [unwired: 7 in]
            }
          }
          n2009 = Boolean Array To Number(Boolean array=w5532) -> (number=w5530:u32)
          n2010 = Max & Min(x=w5527, y=w5526) -> (max(x,y)=w5544:u32)  [unwired: 1 out]
          n2011 = Max & Min(x=w5538, y=w5541) -> (max(x,y)=w5551:u32)  [unwired: 1 out]
          n2012 = Compound Arithmetic op=AND(w5553, w5549, w5547, w5546) -> (w5531:bool)
          n2013 = Max & Min(x=w5552, y=w5551) -> (max(x,y)=w5550:u32)  [unwired: 1 out]
          n2014 = Max & Min(x=w5545, y=w5544) -> (max(x,y)=w5543:u32)  [unwired: 1 out]
          n2015 = case shown="12" w5530 {
            tunnel: w5529 -> [w5600 _ w5612 _ w5621 _ w5627 w5633 _ w5639 w5642 _]
            tunnel: w5526 -> [w5599 w5603 w5608 w5615 w5616 w5624 w5626 _ _ _ _ _]
            tunnel: w5528 -> [w5598 w5601 _ _ w5620 w5622 _ w5632 w5636 _ w5641 _]
            tunnel: w5527 -> [w5597 w5602 w5607 w5613 _ _ _ w5631 w5635 w5638 _ _]
            tunnel: [w5593 w5604 w5609 w5614 w5617 w5623 w5625 w5628 w5634 w5637 w5640 TRUE] -> _
            frame 15 {
              # "A,B,C,D ativos"
              n2016 = Equal?(x=w5600, y=w5598) -> (x = y?=w5596:bool)
              n2017 = Equal?(x=w5597, y=w5599) -> (x = y?=w5594:bool)
              n2018 = Equal?(x=w5598, y=w5597) -> (x = y?=w5595:bool)
              n2019 = Compound Arithmetic op=AND(w5596, w5595, w5594) -> (w5593:bool)
            }
            frame 14 {
              # "B,C e,D ativos"
              n2020 = Equal?(x=w5601, y=w5602) -> (x = y?=w5606:bool)
              n2021 = Equal?(x=w5602, y=w5603) -> (x = y?=w5605:bool)
              n2022 = Compound Arithmetic op=AND(w5606, w5605) -> (w5604:bool)
            }
            frame 13 {
              # "A,C e,D ativos"
              n2023 = Equal?(x=w5612, y=w5607) -> (x = y?=w5611:bool)
              n2024 = Equal?(x=w5607, y=w5608) -> (x = y?=w5610:bool)
              n2025 = Compound Arithmetic op=AND(w5611, w5610) -> (w5609:bool)
            }
            frame 12 {
              # "Só C e D ativos"
              n2026 = Equal?(x=w5613, y=w5615) -> (x = y?=w5614:bool)
            }
            frame 11 {
              # "A,B e,D ativos"
              n2027 = Equal?(x=w5621, y=w5620) -> (x = y?=w5619:bool)
              n2028 = Equal?(x=w5620, y=w5616) -> (x = y?=w5618:bool)
              n2029 = Compound Arithmetic op=AND(w5619, w5618) -> (w5617:bool)
            }
            frame 10 {
              # "Só B e D ativos"
              n2030 = Equal?(x=w5622, y=w5624) -> (x = y?=w5623:bool)
            }
            frame 9 {
              # "Só A e D ativos"
              n2031 = Equal?(x=w5627, y=w5626) -> (x = y?=w5625:bool)
            }
            frame 7 {
              # "A,B,C ativos"
              n2032 = Equal?(x=w5633, y=w5632) -> (x = y?=w5630:bool)
              n2033 = Equal?(x=w5632, y=w5631) -> (x = y?=w5629:bool)
              n2034 = Compound Arithmetic op=AND(w5630, w5629) -> (w5628:bool)
            }
            frame 6 {
              # "Só B e C ativos"
              n2035 = Equal?(x=w5636, y=w5635) -> (x = y?=w5634:bool)
            }
            frame 5 {
              # "Só A e C ativos"
              n2036 = Equal?(x=w5639, y=w5638) -> (x = y?=w5637:bool)
            }
            frame 3 {
              # "só A e B ativos"
              n2037 = Equal?(x=w5642, y=w5641) -> (x = y?=w5640:bool)
            }
            frame 0..2, 4, 8, Default {
              # "nenhum ou só 1  \ncanal ativo."
            }
          }
          n2038 = Compound Arithmetic op=OR(w5525, w5524, w5523, w5522) -> (w5521:bool)
          n2039 = case shown="0..2, 4, 8, Default" w5530 {
            tunnel: w5542 -> [w5651 _ w5663 _ w5672 _ w5678 w5684 _ w5690 w5693 _]
            tunnel: w5541 -> [w5650 w5654 w5659 w5666 w5667 w5675 w5677 _ _ _ _ _]
            tunnel: w5539 -> [w5649 w5652 _ _ w5671 w5673 _ w5683 w5687 _ w5692 _]
            tunnel: w5538 -> [w5648 w5653 w5658 w5664 _ _ _ w5682 w5686 w5689 _ _]
            tunnel: [w5644 w5655 w5660 w5665 w5668 w5674 w5676 w5679 w5685 w5688 w5691 TRUE] -> w5537
            frame 15 {
              # "A,B,C,D ativos"
              n2040 = Equal?(x=w5651, y=w5649) -> (x = y?=w5647:bool)
              n2041 = Equal?(x=w5648, y=w5650) -> (x = y?=w5645:bool)
              n2042 = Equal?(x=w5649, y=w5648) -> (x = y?=w5646:bool)
              n2043 = Compound Arithmetic op=AND(w5647, w5646, w5645) -> (w5644:bool)
            }
            frame 14 {
              # "B,C e,D ativos"
              n2044 = Equal?(x=w5652, y=w5653) -> (x = y?=w5657:bool)
              n2045 = Equal?(x=w5653, y=w5654) -> (x = y?=w5656:bool)
              n2046 = Compound Arithmetic op=AND(w5657, w5656) -> (w5655:bool)
            }
            frame 13 {
              # "A,C e,D ativos"
              n2047 = Equal?(x=w5663, y=w5658) -> (x = y?=w5662:bool)
              n2048 = Equal?(x=w5658, y=w5659) -> (x = y?=w5661:bool)
              n2049 = Compound Arithmetic op=AND(w5662, w5661) -> (w5660:bool)
            }
            frame 12 {
              # "Só C e D ativos"
              n2050 = Equal?(x=w5664, y=w5666) -> (x = y?=w5665:bool)
            }
            frame 11 {
              # "A,B e,D ativos"
              n2051 = Equal?(x=w5672, y=w5671) -> (x = y?=w5670:bool)
              n2052 = Equal?(x=w5671, y=w5667) -> (x = y?=w5669:bool)
              n2053 = Compound Arithmetic op=AND(w5670, w5669) -> (w5668:bool)
            }
            frame 10 {
              # "Só B e D ativos"
              n2054 = Equal?(x=w5673, y=w5675) -> (x = y?=w5674:bool)
            }
            frame 9 {
              # "Só A e D ativos"
              n2055 = Equal?(x=w5678, y=w5677) -> (x = y?=w5676:bool)
            }
            frame 7 {
              # "A,B,C ativos"
              n2056 = Equal?(x=w5684, y=w5683) -> (x = y?=w5681:bool)
              n2057 = Equal?(x=w5683, y=w5682) -> (x = y?=w5680:bool)
              n2058 = Compound Arithmetic op=AND(w5681, w5680) -> (w5679:bool)
            }
            frame 6 {
              # "Só B e C ativos"
              n2059 = Equal?(x=w5687, y=w5686) -> (x = y?=w5685:bool)
            }
            frame 5 {
              # "Só A e C ativos"
              n2060 = Equal?(x=w5690, y=w5689) -> (x = y?=w5688:bool)
            }
            frame 3 {
              # "só A e B ativos"
              n2061 = Equal?(x=w5693, y=w5692) -> (x = y?=w5691:bool)
            }
            frame 0..2, 4, 8, Default {
              # "nenhum ou só 1  \ncanal ativo."
            }
          }
          n2062 = call-dynamic "Write AcquisitionD.vi"("error in (no error)"=w5581, "Acquisition.lvclass"=w5582, "S4ACS_GUI in"=w5580) -> ("error out"=w5571:errorcluster, "S4ACS_GUI out"=w5572:refnum<class "S4GUI.lvclass">)  [unwired: 7 in]
          n2063 = And(x=w5531, y=w5537) -> (x .and. y?=w5540:bool)
          n2064 = case shown="True" w5540 {
            tunnel: w5572 -> [w5696 w5708]
            tunnel: [w5695 w5707] -> w5588
            tunnel: w5550 -> [_ w5706]
            tunnel: w5543 -> [_ _]
            tunnel: w5531 -> [w5697 _]
            tunnel: TRUE -> [_ w5705]
            tunnel: w5521 -> [_ w5704]
            tunnel: w5519 -> [_ w5703]
            frame False {
              n2065 = case shown="True" w5697 {
                tunnel: w5696 -> [w5698 w5702]
                tunnel: [w5698 w5701] -> w5695
                frame False {
                }
                frame True {
                  n2066 = Bundle By Name(cluster=w5702, "Obs_state"=u32 1, "Error Msg"="ERROR: Sequence_done not equal in all active channels.") -> (w5701:refnum<class "S4GUI.lvclass">)
                }
              }
            }
            frame True {
              n2067 = case shown="True" w5705 {
                tunnel: w5708 -> [w5710 w5720]
                tunnel: [w5709 w5719] -> w5707
                tunnel: w5706 -> [_ w5718]
                tunnel: w5704 -> [_ w5714]
                tunnel: w5703 -> [_ w5713]
                frame False {
                  n2068 = Bundle By Name(cluster=w5710, "Obs_state"=u32 1, "Error Msg"="ERROR: Cycles_done not equal in all active channels.") -> (w5709:refnum<class "S4GUI.lvclass">)
                }
                frame True {
                  # "STOP?"
                  n2069 = local read "time308"() -> (w5716:u32)
                  n2070 = Tick Count (ms)() -> (millisecond timer value=w5717:u32)
                  n2071 = Subtract(x=w5717, y=w5716) -> (x-y=→"delay Acq 2":u32)
                  n2072 = case shown="False" w5714 {
                    tunnel: w5720 -> [w5724 w5729]
                    tunnel: [w5723 w5728] -> w5719
                    tunnel: w5718 -> [w5721 w5725]
                    tunnel: w5713 -> [_ w5727]
                    frame True {
                      n2073 = Bundle By Name(cluster=w5724, "Obs_state"=u32 0, "sequesDone"=w5721, "cyclesDone"=w5721) -> (w5723:refnum<class "S4GUI.lvclass">)
                    }
                    frame False {
                      n2074 = Increment(x=w5727) -> (x+1=w5726:u32)
                      n2075 = Bundle By Name(cluster=w5729, "Obs_state"=w5726, "sequesDone"=w5725, "cyclesDone"=w5725) -> (w5728:refnum<class "S4GUI.lvclass">)
                    }
                  }
                }
              }
            }
          }
        }
        frame 368 {
          n2076 = Unbundle By Name(w5831) -> ("TelFocus.lvclass"=w5830:refnum<class "TelFocus.lvclass">)
          n2077 = call-dynamic "VerifSteps.vi"("error in (no error)"=w5827, "TelFocus in"=w5830) -> ("error out"=w5826:errorcluster, "continua?"=w5832:bool, "TelFocus out"=w5829:refnum<class "TelFocus.lvclass">)  [unwired: 7 in]
          n2078 = Bundle By Name(cluster=w5831, "TelFocus.lvclass"=w5829) -> (w5828:refnum<class "S4GUI.lvclass">)
          n2079 = Select(t=u32 360, s=w5832, f=u32 0) -> (s? t:f=w5835:u32)
          n2080 = Bundle By Name(cluster=w5828, "Obs_state"=w5835) -> (w5836:refnum<class "S4GUI.lvclass">)
        }
        frame 400 {
          # "Estado de \"Pause\": fica parado aqui até o botão START seja pressionado."
        }
        frame 500 {
          # "Espera terminar o envio de RESUME para todos os ACS."
          # "Estado de \"Pause\": fica parado aqui até o botão START seja pressionado."
          n2081 = call-dynamic "VerifyAcqIdle.vi"("error in (no error)"=w5841, "S4GUI in"=w5845) -> ("error out"=w5840:errorcluster, "idle"=w5844:bool, "S4GUI out"=w5843:refnum<class "S4GUI.lvclass">)  [unwired: 7 in]
          n2082 = case shown="True" w5844 {
            tunnel: w5843 -> [w5847 w5857]
            tunnel: [w5847 w5849] -> w5842
            tunnel: w5840 -> [w5846 w5856]
            tunnel: [w5846 w5850] -> w5839
            frame False {
            }
            frame True {
              n2083 = call-dynamic "LoadPrevAcqRunState.vi"("error in (no error)"=w5856, "S4GUI in"=w5857) -> ("error out"=w5851:errorcluster, "S4GUI out"=w5852:refnum<class "S4GUI.lvclass">)  [unwired: 8 in]
              n2084 = Tick Count (ms)() -> (millisecond timer value=w5848:u32)
              n2085 = call-dynamic "Read Obs_prevstate.vi"("error in (no error)"=w5851, "S4ACS_GUI in"=w5852) -> ("error out"=w5855:errorcluster, "Obs_prevstate"=w5853:u32, "S4ACS_GUI out"=w5854:refnum<class "S4GUI.lvclass">)  [unwired: 7 in]
              n2086 = local write "time307"(w5848) -> ()
              n2087 = local write "time1"(w5848) -> ()
              n2088 = call-dynamic "Write Obs_state.vi"("error in (no error)"=w5855, "Obs_state"=w5853, "S4ACS_GUI in"=w5854) -> ("error out"=w5850:errorcluster, "S4ACS_GUI out"=w5849:refnum<class "S4GUI.lvclass">)  [unwired: 7 in]
            }
          }
        }
      }
    }
    frame Error {
    }
  }
  "error out" <- w3
  "S4GUI out" <- w2
